vi "Serial Daemon.vi"(8 "UUID":string, 9 "Data Model":refnum<class "Device Data Model.lvclass">, 11 "serial slave":refnum<class "Serial Slave.lvclass">) -> ()   [LabVIEW 2021, in "Serial Slave.lvclass"]
uses:
  Serial Slave.lvclass
  D:/my_projects/projects/Algorithms/Labview/21/Modbus_v121c/Network Protocol/Network Slave/Network Slave.lvclass
  Data Model/Device Data Model.lvclass
  daemon status.ctl
  Transmission Data Unit/Serial Interface/Serial Data Unit.lvclass
  Network Slave.lvclass/Network Slave.ctl
  Serial Slave.lvclass/Serial Slave.ctl
  Transmission Data Unit/Serial Interface/Serial Data Unit.lvclass/Serial Data Unit.ctl
  <vilib>/Instr/_visa.llb/VISA Flush IO Buffer Mask.ctl
  Network Slave.lvclass
panel:
  in  "stop":bool
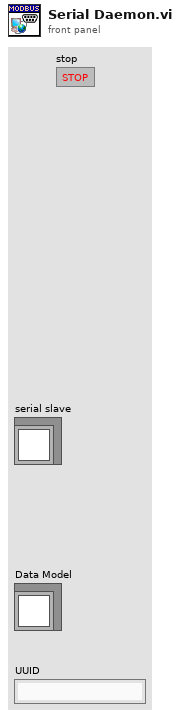
[diagram p1: front panel]
types:
  T1 = typedef "Network Slave.lvclass/daemon status.ctl" = enum16{"Not Started", "Running", "Error", "Stopped"}
  T2 = typedef "VISA Flush IO Buffer Mask.ctl" = u16
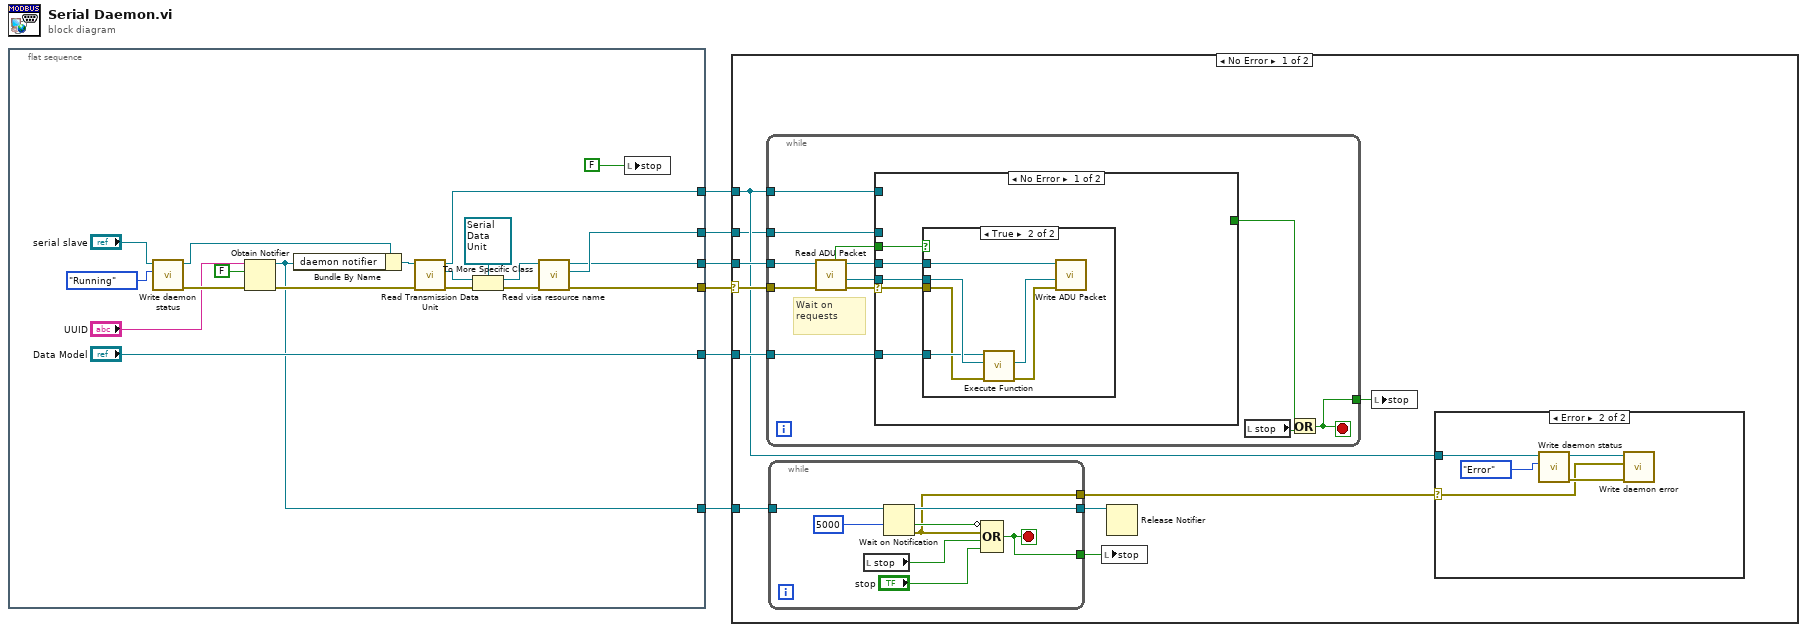
[diagram p0: block diagram]
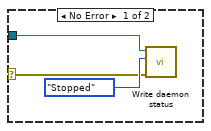
[diagram p2: hidden frame]
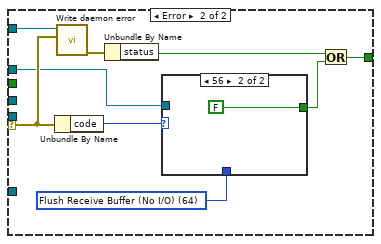
[diagram p4: hidden frame]
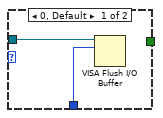
[diagram p5: hidden frame]
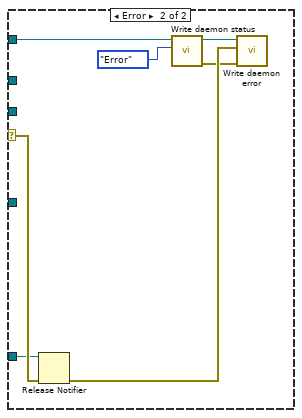
[diagram p6: hidden frame]
diagram:
  n1 = flat-sequence {
    tunnel: [w10] -> w6
    tunnel: ["Data Model"] -> w5
    tunnel: [w9] -> w4
    tunnel: [w12] -> w3
    tunnel: [w17] -> w2
    tunnel: [w13] -> w1
    frame #0 {
      n2 = call "Write daemon status.vi"("daemon status"=daemon_status."Running", "Network Slave in"="serial slave") -> ("error out"=w23:errorcluster, "Network Slave out"=w20:refnum<class "Serial Slave.lvclass">)  [unwired: 8 in]
      n3 = Obtain Notifier(name (unnamed)="UUID", notification data type=FALSE, error in (no error)=w23) -> (notifier out=w12:refnum<notifier>, error out=w21:errorcluster)  [unwired: 1 in, 1 out]
      n4 = Bundle By Name(cluster=w20, "daemon notifier"=w12) -> (w19:refnum<class "Serial Slave.lvclass">)
      n5 = call "Read Transmission Data Unit.vi"("error in (no error)"=w21, "Network Slave in"=w19) -> ("error out"=w7:errorcluster, "Transmission Data Unit"=w8:refnum<class "Transmission Data Unit.lvclass">, "Network Slave out"=w17:refnum<class "Serial Slave.lvclass">)  [unwired: 7 in]
      n6 = To More Specific Class(target class=refnum<class "Serial Data Unit.lvclass"> refnum ("Serial Data Unit"), reference=w8, error in=w7) -> (specific class reference=w15:refnum<class "Serial Data Unit.lvclass">, error out=w16:errorcluster)
      n7 = call "Read visa resource name.vi"("error in (no error)"=w16, "Serial Data Unit in"=w15) -> ("error out"=w9:errorcluster, "visa resource name"=w13:refnum<visa-resource-name>, "Serial Data Unit out"=w10:refnum<class "Serial Data Unit.lvclass">)  [unwired: 7 in]
      n8 = local write "stop"(FALSE ("stop")) -> ()
    }
  }
  n9 = case shown="No Error" w4 {
    selector: w4 -> [w29 w94]
    tunnel: w6 -> [w33 _]
    tunnel: w5 -> [w36 _]
    tunnel: w3 -> [w35 w93]
    tunnel: w2 -> [w28 w88]
    tunnel: w1 -> [w27 _]
    frame No Error {
      n10 = while {
        tunnel: w33 -> [w64]
        tunnel: w36 -> [w62]
        tunnel: w28 -> [w56]
        tunnel: [w59] -> w32
        tunnel: w29 -> [w54]
        tunnel: w27 -> [w53]
        stop <- w59 stop-if-true
        # "Wait on requests"
        n11 = call-dynamic "Read ADU Packet.vi"("error in"=w54, "transmission data unit in"=w64) -> ("error out"=w63:errorcluster, "modbus data unit"=w57:refnum<class "Modbus Data Unit.lvclass">, "transmission data unit out"=w61:refnum<class "Serial Data Unit.lvclass">, "PDU Valid?"=w55:bool)  [unwired: 6 in]
        n12 = case shown="No Error" w63 {
          selector: w63 -> [w66 w78]
          tunnel: w62 -> [w67 _]
          tunnel: w61 -> [w69 _]
          tunnel: [_ w81] -> w58
          tunnel: w57 -> [w68 _]
          tunnel: w56 -> [_ w79]
          tunnel: w55 -> [w65 _]
          tunnel: w53 -> [_ w76]
          frame No Error {
            n13 = case shown="True" w65 {
              tunnel: w69 -> [_ w75]
              tunnel: w68 -> [_ w74]
              tunnel: w67 -> [_ w71]
              tunnel: w66 -> [_ w70]
              frame False {
              }
              frame True {
                n14 = call-dynamic "Execute Function.vi"("error in"=w70, "modbus request"=w74, "device data model in"=w71) -> ("error out"=w72:errorcluster, "modbus response"=w73:refnum<class "Modbus Data Unit.lvclass">)  [unwired: 6 in, 1 out]
                n15 = call-dynamic "Write ADU Packet.vi"("error in"=w72, "modbus data unit"=w73, "transmission data unit in"=w75) -> ()  [unwired: 7 in, 2 out]
              }
            }
          }
          frame Error {
            w83 = T2 64 items=["Flush Receive Buffer"=16, "Write Transmit Buffer to Device"=32, "Flush Receive Buffer (No I/O)"=64, "Flush Transmit Buffer"=128] ("Mask")
            n16 = Unbundle By Name(w78) -> ("code"=w84:i32)
            n17 = call "Write daemon error.vi"("daemon error"=w78, "Network Slave in"=w79) -> ("error out"=w77:errorcluster)  [unwired: 8 in, 1 out]
            n18 = Unbundle By Name(w77) -> ("status"=w80:bool)
            n19 = case shown="56" w84 {
              tunnel: [_ FALSE ("stop")] -> w82
              tunnel: w76 -> [w86 _]
              tunnel: w83 -> [w85 _]
              frame 0, Default {
                n20 = VISA Flush I/O Buffer(VISA resource name=w86, mask (16)=w85) -> ()  [unwired: 1 in, 2 out]
              }
              frame 56 {
              }
            }
            n21 = Or(x=w80, y=w82) -> (x .or. y?=w81:bool)
          }
        }
        n22 = local read "stop"() -> (w60:bool)
        n23 = Or(x=w58, y=w60) -> (x .or. y?=w59:bool)
      }
      n24 = while {
        tunnel: w35 -> [w51]
        tunnel: [w50] -> w34
        tunnel: [w47] -> w30
        tunnel: [w46] -> w31
        stop <- w47 stop-if-true
        n25 = local read "stop"() -> (w48:bool)
        n26 = Wait on Notification(notifier=w51, timeout in ms (-1)=5000) -> (notifier out=w50:refnum<notifier>, timed out?=w49:bool, error out=w46:errorcluster)  [unwired: 2 in, 1 out]
        n27 = Compound Arithmetic op=OR(invert w49, w46, w48, "stop") -> (w47:bool)
      }
      n28 = local write "stop"(w30) -> ()
      n29 = Release Notifier(notifier=w34) -> ()  [unwired: 2 in, 3 out]
      n30 = local write "stop"(w32) -> ()
      n31 = case shown="Error" w31 {
        selector: w31 -> [w38 w40]
        tunnel: w28 -> [w37 w42]
        frame No Error {
          n32 = call "Write daemon status.vi"("error in (no error)"=w38, "daemon status"=daemon_status."Stopped", "Network Slave in"=w37) -> ()  [unwired: 7 in, 2 out]
        }
        frame Error {
          n33 = call "Write daemon status.vi"("daemon status"=daemon_status."Error", "Network Slave in"=w42) -> ("error out"=w43:errorcluster, "Network Slave out"=w44:refnum<class "Serial Slave.lvclass">)  [unwired: 8 in]
          n34 = call "Write daemon error.vi"("error in (no error)"=w43, "daemon error"=w40, "Network Slave in"=w44) -> ()  [unwired: 7 in, 2 out]
        }
      }
    }
    frame Error {
      n35 = Release Notifier(notifier=w93, error in (no error)=w94) -> (error out=w90:errorcluster)  [unwired: 1 in, 2 out]
      n36 = call "Write daemon status.vi"("daemon status"=daemon_status."Error", "Network Slave in"=w88) -> ("error out"=w89:errorcluster, "Network Slave out"=w91:refnum<class "Serial Slave.lvclass">)  [unwired: 8 in]
      n37 = call "Write daemon error.vi"("error in (no error)"=w89, "daemon error"=w90, "Network Slave in"=w91) -> ()  [unwired: 7 in, 2 out]
    }
  }
